vi "Draw parallelity.vi"(0 "Image in":T2, 1 "Arc width":u32=1, 3 "Overlay type":string, 5 "Bounding rectangle array":cluster{"X":dbl, "Y":dbl}[](array[cluster]), 7 "Fixed overlay in":T1, 9 "Size factor":dbl, 11 "error in (no error)":errorcluster, 12 "Overlay color":u32(colorbox)=16711680, 14 "Measurment Name":string) -> (4 "Image Out":T2, 6 "Overlay coordinates":cluster{"X":dbl, "Y":dbl}[](array[cluster]), 15 "error out":errorcluster)   [LabVIEW 2019]
uses:
  <vilib>/vision/Image Controls.llb/IMAQ Image.ctl
  <vilib>/vision/NI_Vision_Development_Module.lvlib
panel:
  in  "Array of input":string[](array[string])
  out "Offset height":dbl
  out "Offset width":dbl
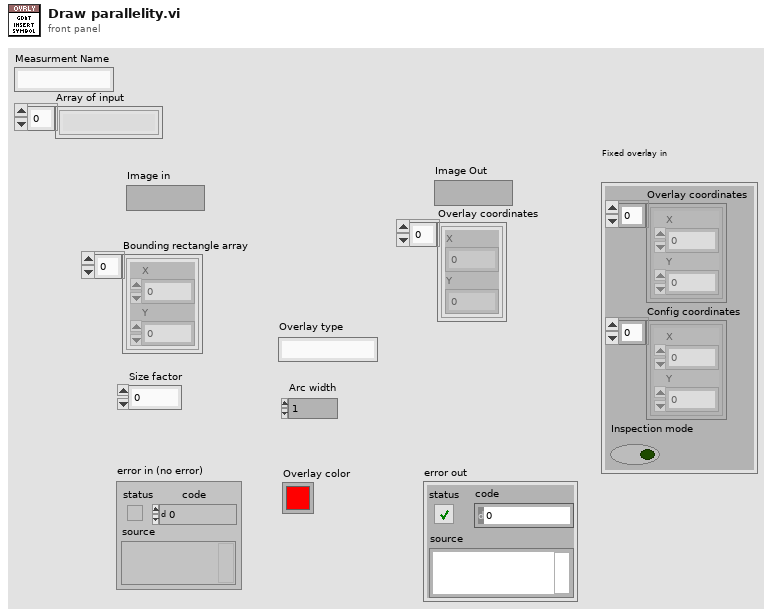
[diagram p1: front panel]
types:
  T1 = cluster{"Overlay coordinates":cluster{"X":dbl, "Y":dbl}[], "Config coordinates":cluster{"X":dbl, "Y":dbl}[], "Inspection mode":bool}
  T2 = typedef "IMAQ Image.ctl" = refnum<image>
  T3 = cluster{"Point 1":cluster{"X":sgl, "Y":sgl}, "Point 2":cluster{"X":sgl, "Y":sgl}}
  T4 = cluster{"Left":i32, "Top":i32, "Right":i32, "Bottom":i32}
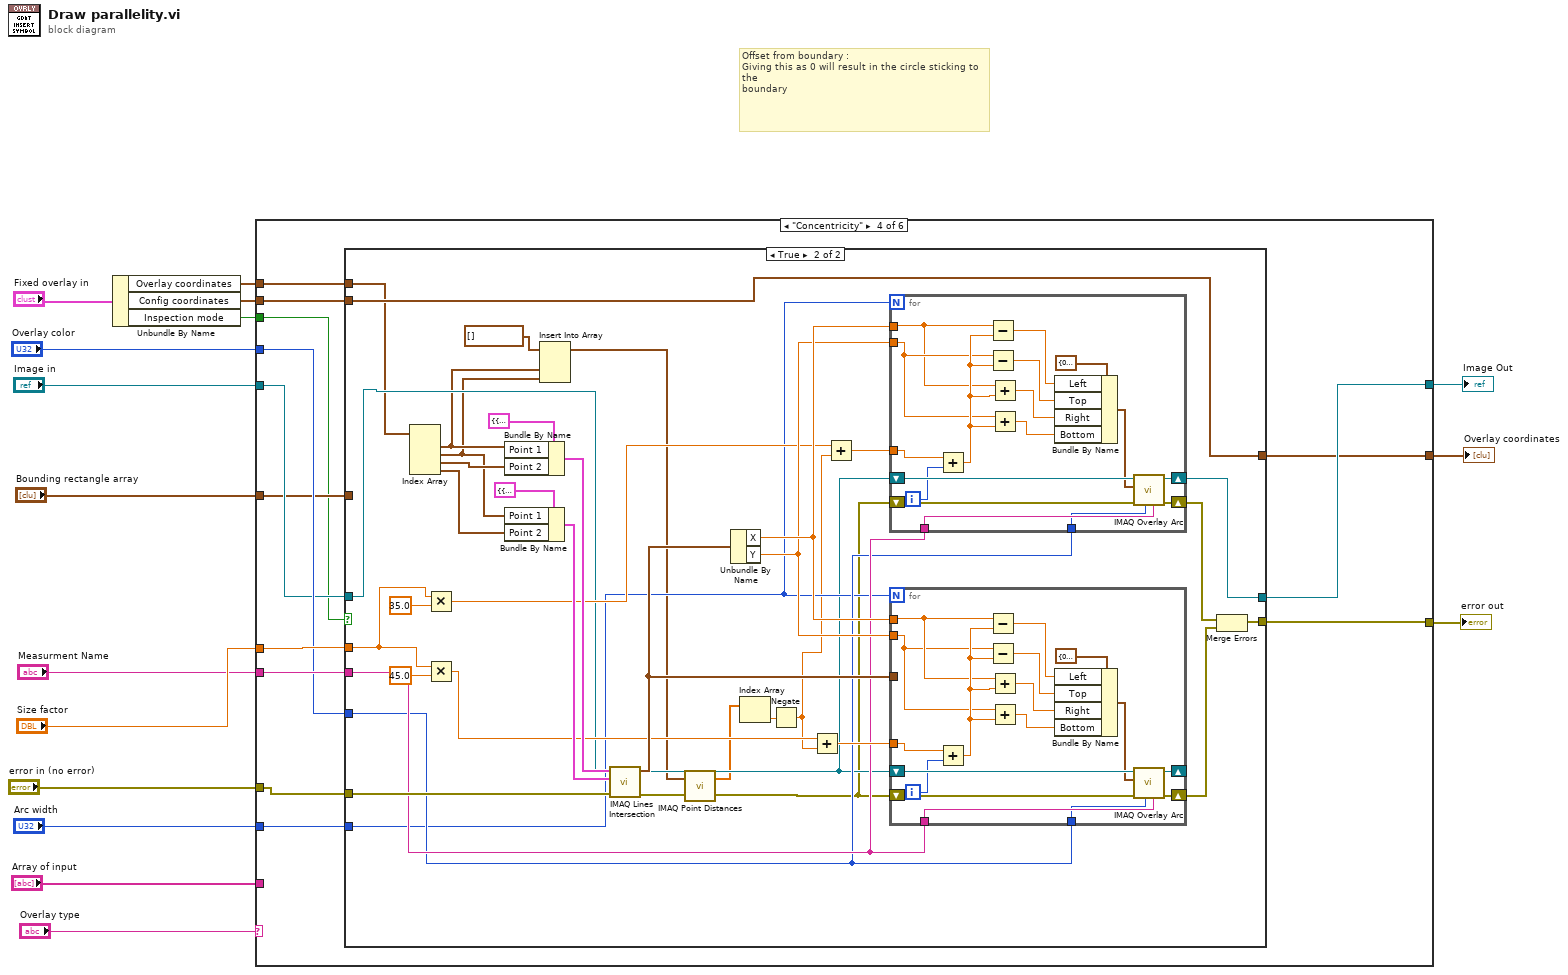
[diagram p0: block diagram]
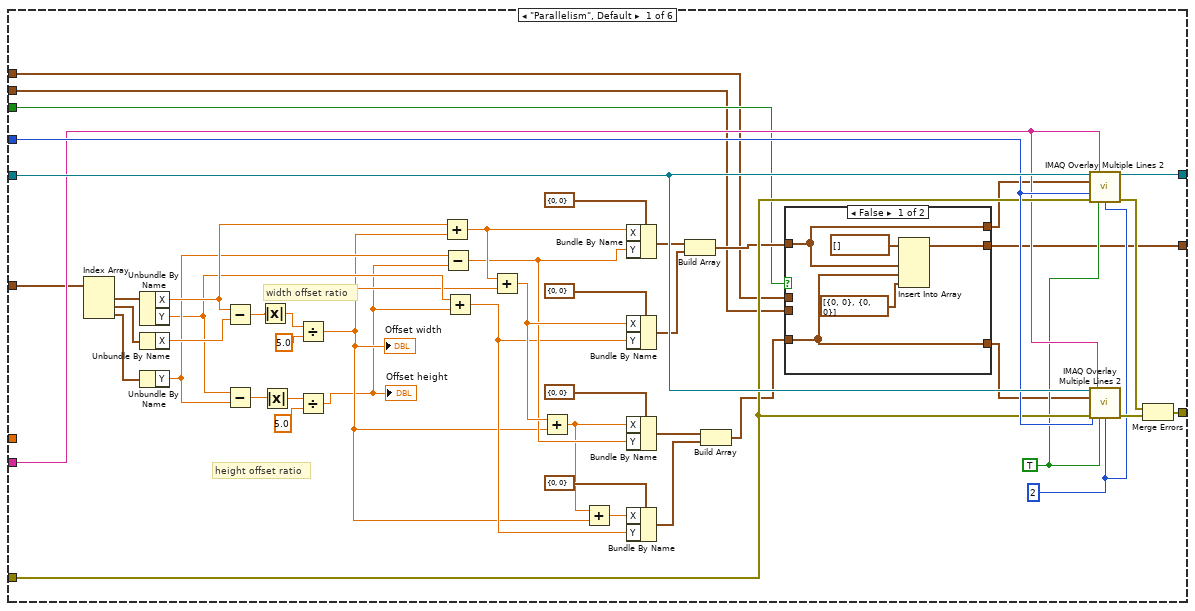
[diagram p2: hidden frame]
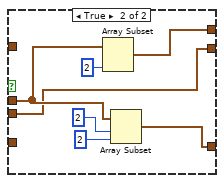
[diagram p3: hidden frame]
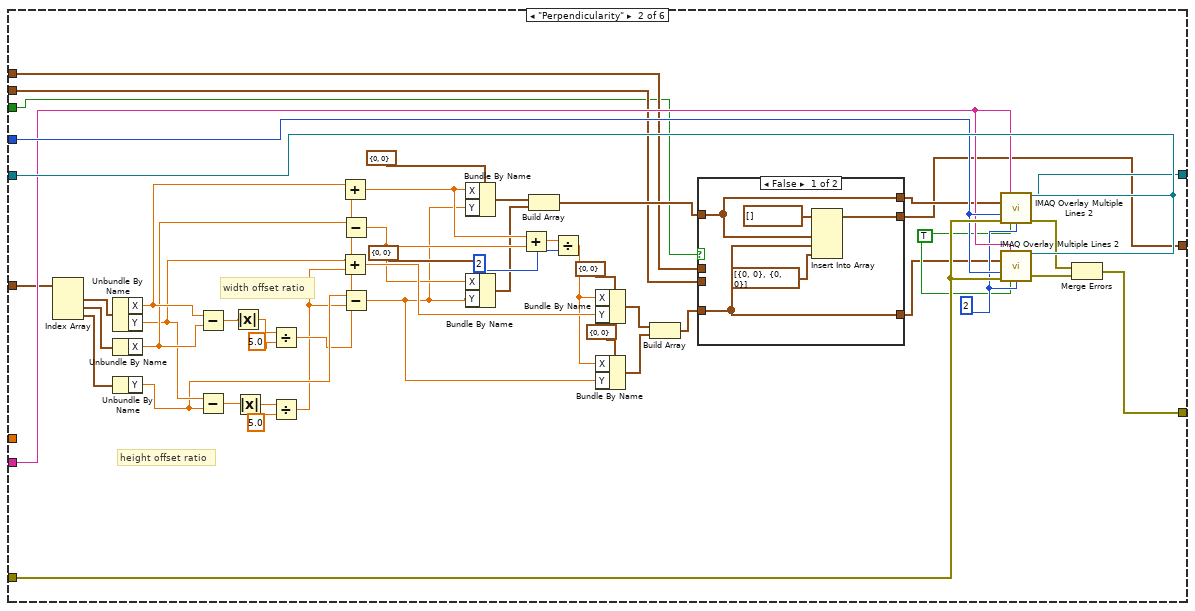
[diagram p4: hidden frame]
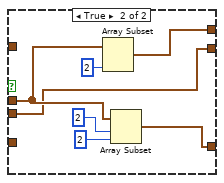
[diagram p5: hidden frame]
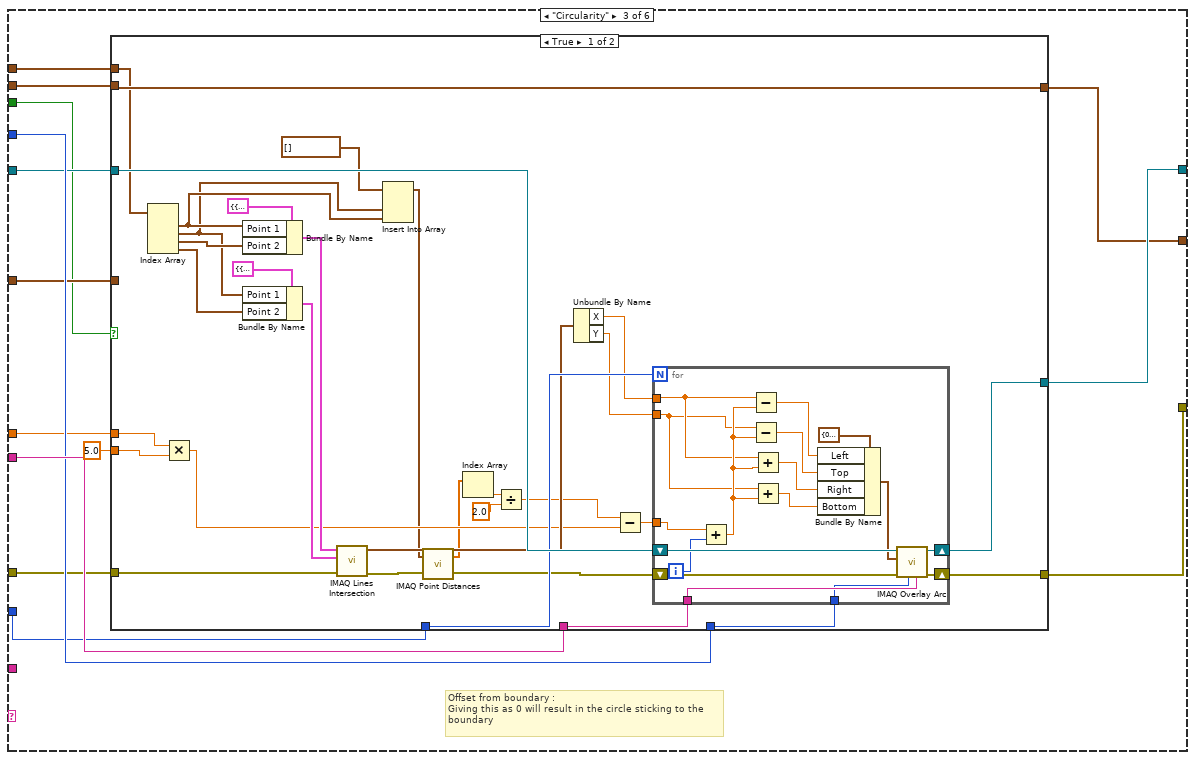
[diagram p6: hidden frame]
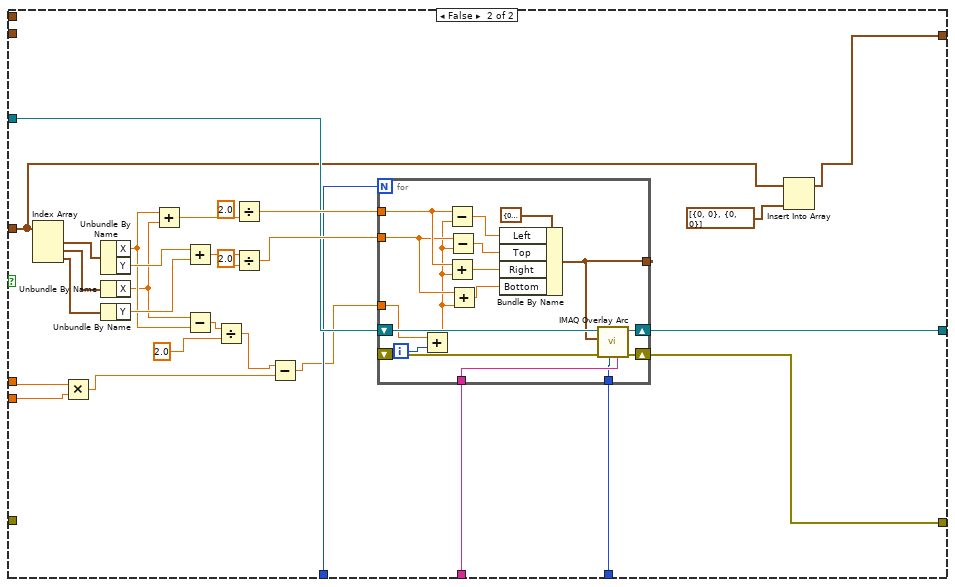
[diagram p7: hidden frame]
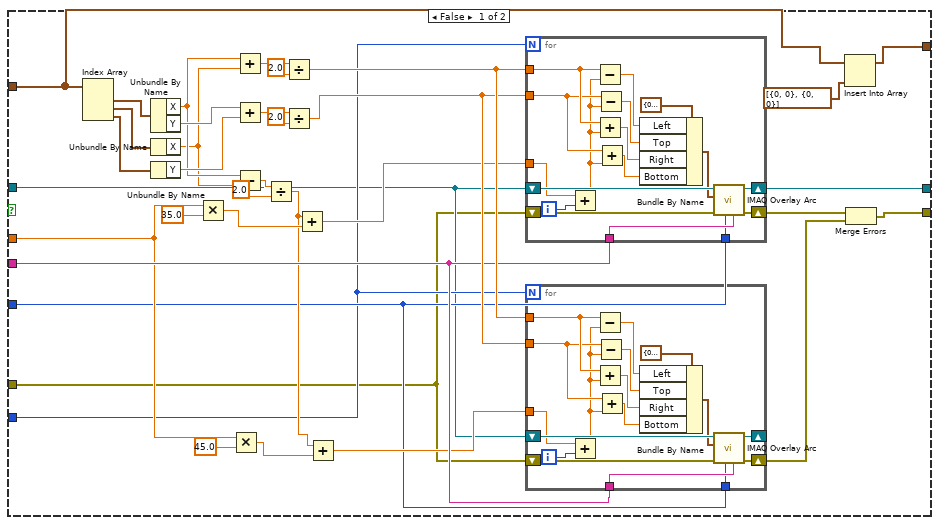
[diagram p8: hidden frame]
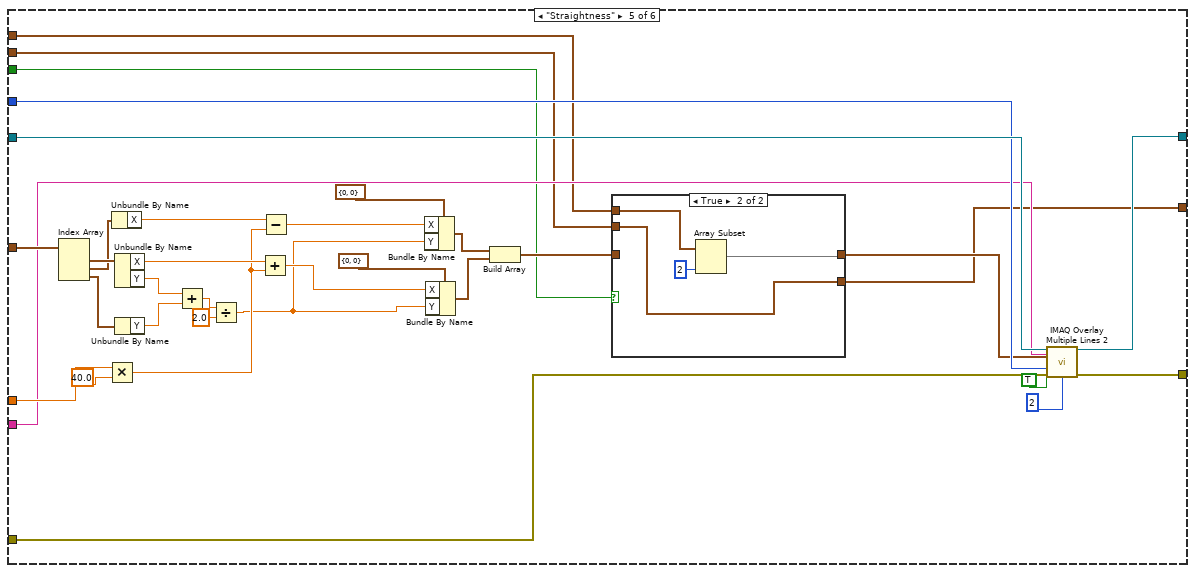
[diagram p9: hidden frame]
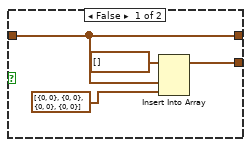
[diagram p10: hidden frame]
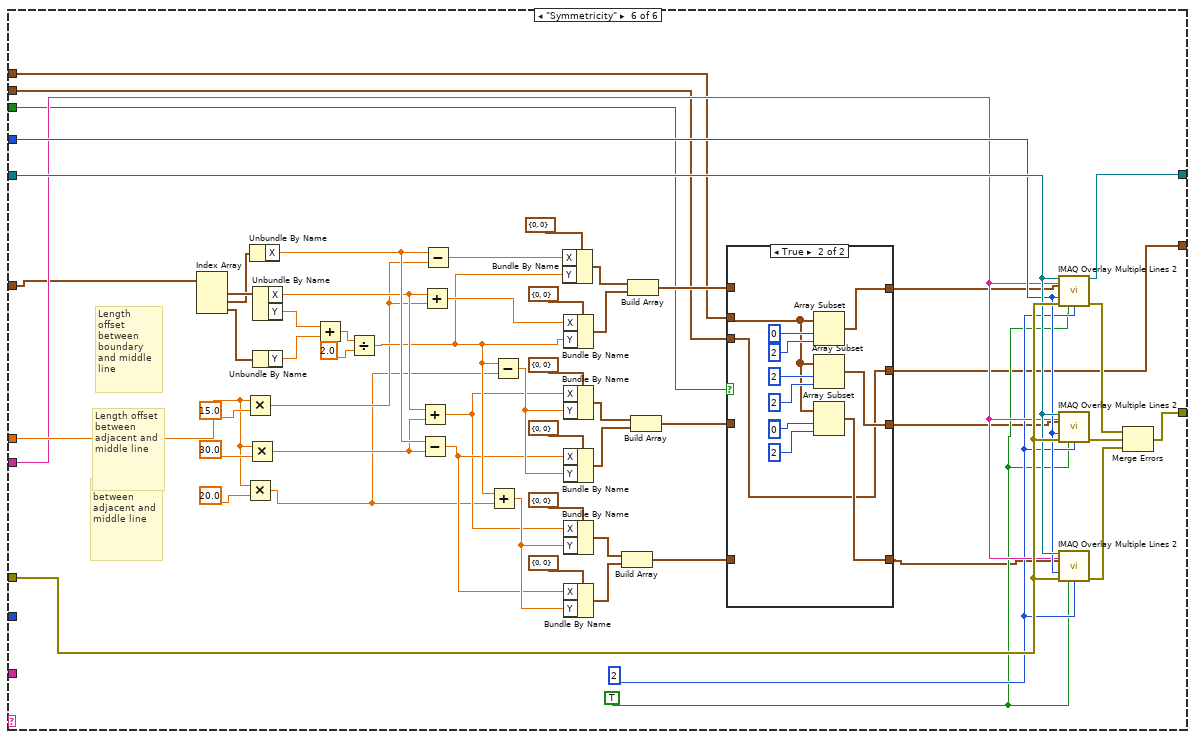
[diagram p11: hidden frame]
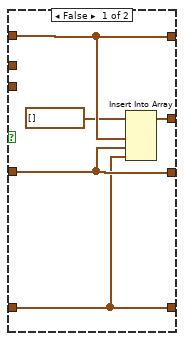
[diagram p12: hidden frame]
diagram:
  # "Offset from boundary :\nGiving this as 0 will result in the circle sticking to the\nboundary"
  n1 = Unbundle By Name("Fixed overlay in") -> ("Overlay coordinates"=w4:cluster{"X":dbl, "Y":dbl}[], "Config coordinates"=w3:cluster{"X":dbl, "Y":dbl}[], "Inspection mode"=w2:bool)
  n2 = case shown="\"Concentricity\"" "Overlay type" {
    tunnel: "Bounding rectangle array" -> [w25 w85 w144 w252 w429 w451]
    tunnel: "Size factor" -> [_ _ w146 w256 w424 w458]
    tunnel: "Image in" -> [w41 w98 w147 w253 w412 w463]
    tunnel: [w38 w94 w149 w259 w409 w455] -> w14
    tunnel: [w37 w93 w148 w258 w408 w483] -> w13
    tunnel: "Overlay color" -> [w36 w92 w150 w255 w411 w462]
    tunnel: "error in (no error)" -> [w31 w97 w140 w251 w410 w464]
    tunnel: "Arc width" -> [_ _ w145 w254 _ _]
    tunnel: "Measurment Name" -> [w28 w88 w151 w257 w407 w454]
    tunnel: "Array of input" -> [_ _ _ _ _ _]
    tunnel: w4 -> [w19 w79 w142 w248 w401 w443]
    tunnel: w3 -> [w18 w78 w143 w250 w400 w442]
    tunnel: w2 -> [w20 w77 w141 w247 w399 w444]
    tunnel: [w17 w80 w139 w249 w402 w441] -> w1
    frame "Parallelism", Default {
      w26 = u32 2 ("Width")
      w27 = TRUE ("Maintain Width?")
      # "height offset ratio"
      # "width offset ratio"
      n3 = Index Array(array=w25) -> (element #1=w64:cluster{"X":dbl, "Y":dbl}, element #2=w63:cluster{"X":dbl, "Y":dbl}, element #3=w58:cluster{"X":dbl, "Y":dbl})  [unwired: 3 in]
      n4 = Unbundle By Name(w64) -> ("X"=w53:dbl, "Y"=w49:dbl)
      n5 = Unbundle By Name(w63) -> ("X"=w62:dbl)
      n6 = Unbundle By Name(w58) -> ("Y"=w52:dbl)
      n7 = Subtract(x=w53, y=w62) -> (x-y=w60:dbl)
      n8 = Subtract(x=w49, y=w52) -> (x-y=w57:dbl)
      n9 = Absolute Value(x=w60) -> (abs(x)=w59:dbl)
      n10 = Absolute Value(x=w57) -> (abs(x)=w56:dbl)
      n11 = Divide(x=w59, y=5.0) -> (x/y=w30:dbl)
      "Offset width" <- w30
      n12 = Divide(x=w56, y=5.0) -> (x/y=w29:dbl)
      "Offset height" <- w29
      n13 = Add(x=w53, y=w30) -> (x+y=w50:dbl)
      n14 = Subtract(x=w52, y=w29) -> (x-y=w45:dbl)
      n15 = Add(x=w49, y=w29) -> (x+y=w42:dbl)
      n16 = Add(x=w50, y=w30) -> (x+y=w46:dbl)
      n17 = Add(x=w46, y=w30) -> (x+y=w43:dbl)
      n18 = Add(x=w43, y=w30) -> (x+y=w44:dbl)
      n19 = Bundle By Name(cluster=cluster{"X":i32, "Y":i32} {"X"=0, "Y"=0} ("Start Point"), "X"=w50, "Y"=w45) -> (w33:cluster{"X":i32, "Y":i32})
      n20 = Bundle By Name(cluster=cluster{"X":i32, "Y":i32} {"X"=0, "Y"=0} ("Start Point"), "X"=w46, "Y"=w42) -> (w32:cluster{"X":i32, "Y":i32})
      n21 = Bundle By Name(cluster=cluster{"X":i32, "Y":i32} {"X"=0, "Y"=0} ("Start Point"), "X"=w43, "Y"=w45) -> (w35:cluster{"X":i32, "Y":i32})
      n22 = Bundle By Name(cluster=cluster{"X":i32, "Y":i32} {"X"=0, "Y"=0} ("Start Point"), "X"=w44, "Y"=w42) -> (w34:cluster{"X":i32, "Y":i32})
      n23 = Build Array(w33, w32) -> (w24:cluster{"X":i32, "Y":i32}[])
      n24 = Build Array(w35, w34) -> (w22:cluster{"X":i32, "Y":i32}[])
      n25 = case shown="False" w20 {
        tunnel: w24 -> [w68 _]
        tunnel: w22 -> [w66 _]
        tunnel: [w68 w73] -> w23
        tunnel: [w67 w70] -> w17
        tunnel: [w66 w72] -> w21
        tunnel: w19 -> [_ w71]
        tunnel: w18 -> [_ w70]
        frame False {
          n26 = Insert Into Array(array=cluster{"X":i32, "Y":i32}[] [], new element #1=w68, new element #2=w66, new element #3=cluster{"X":i32, "Y":i32}[] [{"X"=0, "Y"=0}, {"X"=0, "Y"=0}]) -> (w67:cluster{"X":i32, "Y":i32}[])  [unwired: 1 in]
        }
        frame True {
          n27 = Array Subset(array=w71, length=2) -> (w73:cluster{"X":dbl, "Y":dbl}[])  [unwired: 1 in]
          n28 = Array Subset(array=w71, index=2 ("length"), length=2) -> (w72:cluster{"X":dbl, "Y":dbl}[])
        }
      }
      n29 = call "IMAQ Overlay Multiple Lines 2"("Image"=w41, "Group"=w28, "Line End Points"=w23, "Color"=w36, "error in (no error)"=w31, "Maintain Width?"=w27, "Width"=w26) -> ("Image Out"=w37:T2, "error out"=w40:errorcluster)  [unwired: 7 in]
      n30 = call "IMAQ Overlay Multiple Lines 2"("Image"=w41, "Group"=w28, "Line End Points"=w21, "Color"=w36, "error in (no error)"=w31, "Maintain Width?"=w27, "Width"=w26) -> ("error out"=w39:errorcluster)  [unwired: 7 in, 1 out]
      n31 = Merge Errors(w40, w39) -> (w38:errorcluster)
    }
    frame "Perpendicularity" {
      w87 = u32 2 ("Width")
      w86 = TRUE ("Maintain Width?")
      # "height offset ratio"
      # "width offset ratio"
      n32 = Index Array(array=w85) -> (element #1=w119:cluster{"X":dbl, "Y":dbl}, element #2=w118:cluster{"X":dbl, "Y":dbl}, element #3=w117:cluster{"X":dbl, "Y":dbl})  [unwired: 3 in]
      n33 = Unbundle By Name(w119) -> ("X"=w116:dbl, "Y"=w114:dbl)
      n34 = Unbundle By Name(w118) -> ("X"=w115:dbl)
      n35 = Unbundle By Name(w117) -> ("Y"=w91:dbl)
      n36 = Subtract(x=w116, y=w115) -> (x-y=w124:dbl)
      n37 = Subtract(x=w114, y=w91) -> (x-y=w122:dbl)
      n38 = Absolute Value(x=w124) -> (abs(x)=w123:dbl)
      n39 = Absolute Value(x=w122) -> (abs(x)=w121:dbl)
      n40 = Divide(x=w123, y=5.0) -> (x/y=w90:dbl)
      n41 = Divide(x=w121, y=5.0) -> (x/y=w89:dbl)
      n42 = Add(x=w116, y=w90) -> (x+y=w107:dbl)
      n43 = Add(x=w114, y=w89) -> (x+y=w110:dbl)
      n44 = Subtract(x=w115, y=w90) -> (x-y=w106:dbl)
      n45 = Subtract(x=w91, y=w89) -> (x-y=w103:dbl)
      n46 = Bundle By Name(cluster=cluster{"X":i32, "Y":i32} {"X"=0, "Y"=0} ("Start Point"), "X"=w107, "Y"=w103) -> (w102:cluster{"X":i32, "Y":i32})
      n47 = Bundle By Name(cluster=cluster{"X":i32, "Y":i32} {"X"=0, "Y"=0} ("Start Point"), "X"=w106, "Y"=w103) -> (w101:cluster{"X":i32, "Y":i32})
      n48 = Add(x=w107, y=w106) -> (x+y=w109:dbl)
      n49 = Build Array(w102, w101) -> (w82:cluster{"X":i32, "Y":i32}[])
      n50 = Divide(x=w109, y=2) -> (x/y=w104:dbl)
      n51 = Bundle By Name(cluster=cluster{"X":i32, "Y":i32} {"X"=0, "Y"=0} ("Start Point"), "X"=w104, "Y"=w110) -> (w100:cluster{"X":i32, "Y":i32})
      n52 = Bundle By Name(cluster=cluster{"X":i32, "Y":i32} {"X"=0, "Y"=0} ("Start Point"), "X"=w104, "Y"=w103) -> (w99:cluster{"X":i32, "Y":i32})
      n53 = Build Array(w100, w99) -> (w84:cluster{"X":i32, "Y":i32}[])
      n54 = case shown="False" w77 {
        tunnel: w82 -> [w129 _]
        tunnel: w84 -> [w127 _]
        tunnel: [w129 w134] -> w81
        tunnel: [w128 w131] -> w80
        tunnel: [w127 w133] -> w83
        tunnel: w79 -> [_ w132]
        tunnel: w78 -> [_ w131]
        frame False {
          n55 = Insert Into Array(array=cluster{"X":i32, "Y":i32}[] [], new element #1=w129, new element #2=w127, new element #3=cluster{"X":i32, "Y":i32}[] [{"X"=0, "Y"=0}, {"X"=0, "Y"=0}]) -> (w128:cluster{"X":i32, "Y":i32}[])  [unwired: 1 in]
        }
        frame True {
          n56 = Array Subset(array=w132, length=2) -> (w134:cluster{"X":dbl, "Y":dbl}[])  [unwired: 1 in]
          n57 = Array Subset(array=w132, index=2 ("length"), length=2) -> (w133:cluster{"X":dbl, "Y":dbl}[])
        }
      }
      n58 = call "IMAQ Overlay Multiple Lines 2"("Image"=w98, "Group"=w88, "Line End Points"=w81, "Color"=w92, "error in (no error)"=w97, "Maintain Width?"=w86, "Width"=w87) -> ("Image Out"=w93:T2, "error out"=w95:errorcluster)  [unwired: 7 in]
      n59 = call "IMAQ Overlay Multiple Lines 2"("Image"=w98, "Group"=w88, "Line End Points"=w83, "Color"=w92, "error in (no error)"=w97, "Maintain Width?"=w86, "Width"=w87) -> ("error out"=w96:errorcluster)  [unwired: 7 in, 1 out]
      n60 = Merge Errors(w95, w96) -> (w94:errorcluster)
    }
    frame "Circularity" {
      # "Offset from boundary :\nGiving this as 0 will result in the circle sticking to the\nboundary"
      n61 = case shown="True" w141 {
        tunnel: w151 -> [w183 w215]
        tunnel: w150 -> [w182 w214]
        tunnel: [w181 w213] -> w149
        tunnel: [w180 w212] -> w148
        tunnel: w147 -> [w179 w211]
        tunnel: w146 -> [w165 w205]
        tunnel: w145 -> [w178 w209]
        tunnel: w144 -> [_ w207]
        tunnel: [w177 w206] -> w139
        tunnel: w143 -> [w177 _]
        tunnel: w142 -> [w176 _]
        tunnel: w140 -> [w171 _]
        tunnel: 5.0 ("y") -> [w162 w201]
        frame True {
          n62 = Index Array(array=w176) -> (element #1=w160:cluster{"X":dbl, "Y":dbl}, element #2=w159:cluster{"X":dbl, "Y":dbl}, element #3=w173:cluster{"X":dbl, "Y":dbl}, element #4=w172:cluster{"X":dbl, "Y":dbl})  [unwired: 4 in]
          n63 = Multiply(x=w165, y=w162) -> (x*y=w164:dbl)
          n64 = Bundle By Name(cluster=T3 {"Point 1"={"X"=0.0, "Y"=0.0}, "Point 2"={"X"=0.0, "Y"=0.0}} ("Line 1"), "Point 1"=w160, "Point 2"=w173) -> (w170:T3)
          n65 = Bundle By Name(cluster=T3 {"Point 1"={"X"=0.0, "Y"=0.0}, "Point 2"={"X"=0.0, "Y"=0.0}} ("Line 1"), "Point 1"=w159, "Point 2"=w172) -> (w169:T3)
          n66 = call "IMAQ Lines Intersection"("error in (no error)"=w171, "Line 2"=w169, "Line 1"=w170) -> ("error out"=w161:errorcluster, "Intersection Point"=w166:cluster{"X":sgl, "Y":sgl})  [unwired: 6 in, 1 out]
          n67 = Insert Into Array(array=cluster{"X":dbl, "Y":dbl}[] [], new element #1=w159, new element #2=w160) -> (w157:cluster{"X":dbl, "Y":dbl}[])  [unwired: 1 in]
          n68 = call "IMAQ Point Distances"("Points"=w157, "error in (no error)"=w161) -> ("Distances"=w156:sgl[], "error out"=w152:errorcluster)  [unwired: 3 in]
          n69 = Index Array(array=w156) -> (element=w155:sgl)  [unwired: 1 in]
          n70 = Divide(x=w155, y=sgl 2.0) -> (x/y=w153:sgl)
          n71 = Unbundle By Name(w166) -> ("X"=w168:sgl, "Y"=w167:sgl)
          n72 = Subtract(x=w153, y=w164) -> (x-y=w163:dbl)
          n73 = for {
            N: w178 -> [_]
            shift-right: [w199] -> w181
            shift-left: w152 -> [w200]
            shift-right: [w197] -> w180
            shift-left: w179 -> [w198]
            tunnel: w183 -> [w195]
            tunnel: w182 -> [w194]
            tunnel: w168 -> [w185]
            tunnel: w167 -> [w184]
            tunnel: w163 -> [w188]
            i -> [w187]
            n74 = Add(x=w188, y=w187) -> (x+y=w186:dbl)
            n75 = Subtract(x=w185, y=w186) -> (x-y=w192:dbl)
            n76 = Subtract(x=w184, y=w186) -> (x-y=w191:dbl)
            n77 = Add(x=w185, y=w186) -> (x+y=w190:dbl)
            n78 = Add(x=w184, y=w186) -> (x+y=w189:dbl)
            n79 = Bundle By Name(cluster=T4 {"Left"=0, "Top"=0, "Right"=0, "Bottom"=0} ("Bounding Rectangle"), "Left"=w192, "Top"=w191, "Right"=w190, "Bottom"=w189) -> (w193:T4)
            n80 = call "IMAQ Overlay Arc"("Group"=w195, "Color"=w194, "error in (no error)"=w200, "Bounding Rectangle"=w193, "Image"=w198) -> ("error out"=w199:errorcluster, "Image Out"=w197:T2)  [unwired: 5 in]
          }
        }
        frame False {
          n81 = Index Array(array=w207) -> (element #1=w229:cluster{"X":dbl, "Y":dbl}, element #2=w228:cluster{"X":dbl, "Y":dbl}, element #3=w227:cluster{"X":dbl, "Y":dbl})  [unwired: 3 in]
          n82 = Multiply(x=w205, y=w201) -> (x*y=w203:dbl)
          n83 = Unbundle By Name(w229) -> ("X"=w218:dbl, "Y"=w222:dbl)
          n84 = Unbundle By Name(w228) -> ("X"=w217:dbl)
          n85 = Unbundle By Name(w227) -> ("Y"=w221:dbl)
          n86 = Add(x=w218, y=w217) -> (x+y=w226:dbl)
          n87 = Add(x=w222, y=w221) -> (x+y=w223:dbl)
          n88 = Subtract(x=w217, y=w218) -> (x-y=w216:dbl)
          n89 = Divide(x=w216, y=2.0) -> (x/y=w204:dbl)
          n90 = Divide(x=w226, y=2.0) -> (x/y=w220:dbl)
          n91 = Divide(x=w223, y=2.0) -> (x/y=w219:dbl)
          n92 = Subtract(x=w204, y=w203) -> (x-y=w202:dbl)
          n93 = for {
            N: w209 -> [_]
            tunnel: w220 -> [w239]
            tunnel: w219 -> [w237]
            tunnel: w202 -> [w234]
            shift-right: [w245] -> w213
            shift-left: _ -> [w246]
            shift-right: [w243] -> w212
            shift-left: w211 -> [w244]
            tunnel: w215 -> [w232]
            tunnel: w214 -> [w231]
            tunnel: [w230] -> _
            i -> [w235]
            n94 = Add(x=w234, y=w235) -> (x+y=w233:dbl)
            n95 = Subtract(x=w239, y=w233) -> (x-y=w241:dbl)
            n96 = Add(x=w239, y=w233) -> (x+y=w238:dbl)
            n97 = Subtract(x=w237, y=w233) -> (x-y=w240:dbl)
            n98 = Add(x=w237, y=w233) -> (x+y=w236:dbl)
            n99 = Bundle By Name(cluster=T4 {"Left"=0, "Top"=0, "Right"=0, "Bottom"=0} ("Bounding Rectangle"), "Left"=w241, "Top"=w240, "Right"=w238, "Bottom"=w236) -> (w230:T4)
            n100 = call "IMAQ Overlay Arc"("Group"=w232, "Color"=w231, "error in (no error)"=w246, "Bounding Rectangle"=w230, "Image"=w244) -> ("error out"=w245:errorcluster, "Image Out"=w243:T2)  [unwired: 5 in]
          }
          n101 = Insert Into Array(array=w207, new element=cluster{"X":i32, "Y":i32}[] [{"X"=0, "Y"=0}, {"X"=0, "Y"=0}]) -> (w206:cluster{"X":dbl, "Y":dbl}[])  [unwired: 1 in]
        }
      }
    }
    frame "Concentricity" {
      n102 = case shown="True" w247 {
        tunnel: [w264 w354] -> w259
        tunnel: [w282 w341] -> w258
        tunnel: w257 -> [w275 w344]
        tunnel: w256 -> [w272 w347]
        tunnel: w255 -> [w269 w343]
        tunnel: w254 -> [w268 w342]
        tunnel: w253 -> [w267 w340]
        tunnel: w252 -> [w261 _]
        tunnel: w251 -> [w263 w355]
        tunnel: w250 -> [_ w339]
        tunnel: [w260 w339] -> w249
        tunnel: w248 -> [_ w338]
        frame False {
          n103 = Index Array(array=w261) -> (element #1=w294:cluster{"X":dbl, "Y":dbl}, element #2=w293:cluster{"X":dbl, "Y":dbl}, element #3=w292:cluster{"X":dbl, "Y":dbl})  [unwired: 3 in]
          n104 = Unbundle By Name(w294) -> ("X"=w285:dbl, "Y"=w287:dbl)
          n105 = Unbundle By Name(w293) -> ("X"=w284:dbl)
          n106 = Unbundle By Name(w292) -> ("Y"=w286:dbl)
          n107 = Multiply(x=w272, y=35.0) -> (x*y=w279:dbl)
          n108 = Multiply(x=w272, y=45.0) -> (x*y=w271:dbl)
          n109 = Add(x=w285, y=w284) -> (x+y=w291:dbl)
          n110 = Add(x=w287, y=w286) -> (x+y=w288:dbl)
          n111 = Subtract(x=w285, y=w284) -> (x-y=w283:dbl)
          n112 = Divide(x=w283, y=2.0) -> (x/y=w274:dbl)
          n113 = Divide(x=w291, y=2.0) -> (x/y=w278:dbl)
          n114 = Divide(x=w288, y=2.0) -> (x/y=w277:dbl)
          n115 = Add(x=w274, y=w279) -> (x+y=w276:dbl)
          n116 = Add(x=w274, y=w271) -> (x+y=w270:dbl)
          n117 = for {
            N: w268 -> [_]
            tunnel: w278 -> [w320]
            tunnel: w277 -> [w318]
            tunnel: w276 -> [w315]
            shift-right: [w327] -> w266
            shift-left: w263 -> [w328]
            shift-right: [w325] -> w282
            shift-left: w267 -> [w326]
            tunnel: w275 -> [w313]
            tunnel: w269 -> [w312]
            i -> [w316]
            n118 = Add(x=w315, y=w316) -> (x+y=w314:dbl)
            n119 = Subtract(x=w320, y=w314) -> (x-y=w322:dbl)
            n120 = Add(x=w320, y=w314) -> (x+y=w319:dbl)
            n121 = Subtract(x=w318, y=w314) -> (x-y=w321:dbl)
            n122 = Add(x=w318, y=w314) -> (x+y=w317:dbl)
            n123 = Bundle By Name(cluster=T4 {"Left"=0, "Top"=0, "Right"=0, "Bottom"=0} ("Bounding Rectangle"), "Left"=w322, "Top"=w321, "Right"=w319, "Bottom"=w317) -> (w323:T4)
            n124 = call "IMAQ Overlay Arc"("Group"=w313, "Color"=w312, "error in (no error)"=w328, "Bounding Rectangle"=w323, "Image"=w326) -> ("error out"=w327:errorcluster, "Image Out"=w325:T2)  [unwired: 5 in]
          }
          n125 = for {
            N: w268 -> [_]
            tunnel: w278 -> [w303]
            tunnel: w277 -> [w301]
            tunnel: w270 -> [w298]
            shift-right: [w310] -> w265
            shift-left: w263 -> [w311]
            shift-right: [w308] -> _
            shift-left: w267 -> [w309]
            tunnel: w275 -> [w296]
            tunnel: w269 -> [w295]
            i -> [w299]
            n126 = Add(x=w298, y=w299) -> (x+y=w297:dbl)
            n127 = Subtract(x=w303, y=w297) -> (x-y=w305:dbl)
            n128 = Add(x=w303, y=w297) -> (x+y=w302:dbl)
            n129 = Subtract(x=w301, y=w297) -> (x-y=w304:dbl)
            n130 = Add(x=w301, y=w297) -> (x+y=w300:dbl)
            n131 = Bundle By Name(cluster=T4 {"Left"=0, "Top"=0, "Right"=0, "Bottom"=0} ("Bounding Rectangle"), "Left"=w305, "Top"=w304, "Right"=w302, "Bottom"=w300) -> (w306:T4)
            n132 = call "IMAQ Overlay Arc"("Group"=w296, "Color"=w295, "error in (no error)"=w311, "Bounding Rectangle"=w306, "Image"=w309) -> ("error out"=w310:errorcluster, "Image Out"=w308:T2)  [unwired: 5 in]
          }
          n133 = Insert Into Array(array=w261, new element=cluster{"X":i32, "Y":i32}[] [{"X"=0, "Y"=0}, {"X"=0, "Y"=0}]) -> (w260:cluster{"X":dbl, "Y":dbl}[])  [unwired: 1 in]
          n134 = Merge Errors(w266, w265) -> (w264:errorcluster)
        }
        frame True {
          n135 = Index Array(array=w338) -> (element #1=w335:cluster{"X":dbl, "Y":dbl}, element #2=w334:cluster{"X":dbl, "Y":dbl}, element #3=w362:cluster{"X":dbl, "Y":dbl}, element #4=w361:cluster{"X":dbl, "Y":dbl})  [unwired: 4 in]
          n136 = Multiply(x=w347, y=35.0) -> (x*y=w346:dbl)
          n137 = Multiply(x=w347, y=45.0) -> (x*y=w356:dbl)
          n138 = Bundle By Name(cluster=T3 {"Point 1"={"X"=0.0, "Y"=0.0}, "Point 2"={"X"=0.0, "Y"=0.0}} ("Line 1"), "Point 1"=w335, "Point 2"=w362) -> (w360:T3)
          n139 = Bundle By Name(cluster=T3 {"Point 1"={"X"=0.0, "Y"=0.0}, "Point 2"={"X"=0.0, "Y"=0.0}} ("Line 1"), "Point 1"=w334, "Point 2"=w361) -> (w359:T3)
          n140 = Insert Into Array(array=cluster{"X":dbl, "Y":dbl}[] [], new element #1=w335, new element #2=w334) -> (w332:cluster{"X":dbl, "Y":dbl}[])  [unwired: 1 in]
          n141 = call "IMAQ Lines Intersection"("error in (no error)"=w355, "Line 2"=w359, "Line 1"=w360) -> ("error out"=w337:errorcluster, "Intersection Point"=w358:cluster{"X":sgl, "Y":sgl})  [unwired: 6 in, 1 out]
          n142 = call "IMAQ Point Distances"("Points"=w332, "error in (no error)"=w337) -> ("Distances"=w331:sgl[], "error out"=w336:errorcluster)  [unwired: 3 in]
          n143 = Unbundle By Name(w358) -> ("X"=w351:sgl, "Y"=w350:sgl)
          n144 = Index Array(array=w331) -> (element=w330:sgl)  [unwired: 1 in]
          n145 = Negate(x=w330) -> (-x=w329:sgl)
          n146 = Add(x=w356, y=w329) -> (x+y=w349:dbl)
          n147 = Add(x=w346, y=w329) -> (x+y=w345:dbl)
          n148 = for {
            N: w342 -> [_]
            shift-right: [w380] -> w352
            shift-left: w336 -> [w381]
            shift-right: [w378] -> w341
            shift-left: w340 -> [w379]
            tunnel: w344 -> [w376]
            tunnel: w343 -> [w375]
            tunnel: w351 -> [w365]
            tunnel: w350 -> [w366]
            tunnel: w345 -> [w369]
            i -> [w368]
            n149 = Add(x=w369, y=w368) -> (x+y=w367:dbl)
            n150 = Subtract(x=w365, y=w367) -> (x-y=w373:dbl)
            n151 = Subtract(x=w366, y=w367) -> (x-y=w372:dbl)
            n152 = Add(x=w365, y=w367) -> (x+y=w371:dbl)
            n153 = Add(x=w366, y=w367) -> (x+y=w370:dbl)
            n154 = Bundle By Name(cluster=T4 {"Left"=0, "Top"=0, "Right"=0, "Bottom"=0} ("Bounding Rectangle"), "Left"=w373, "Top"=w372, "Right"=w371, "Bottom"=w370) -> (w374:T4)
            n155 = call "IMAQ Overlay Arc"("Group"=w376, "Color"=w375, "error in (no error)"=w381, "Bounding Rectangle"=w374, "Image"=w379) -> ("error out"=w380:errorcluster, "Image Out"=w378:T2)  [unwired: 5 in]
          }
          n156 = for {
            N: w342 -> [_]
            shift-right: [w397] -> w353
            shift-left: w336 -> [w398]
            shift-right: [w395] -> _
            shift-left: w340 -> [w396]
            tunnel: w344 -> [w393]
            tunnel: w343 -> [w392]
            tunnel: w358 -> [_]
            tunnel: w351 -> [w383]
            tunnel: w350 -> [w382]
            tunnel: w349 -> [w386]
            i -> [w385]
            n157 = Add(x=w386, y=w385) -> (x+y=w384:dbl)
            n158 = Subtract(x=w383, y=w384) -> (x-y=w390:dbl)
            n159 = Subtract(x=w382, y=w384) -> (x-y=w389:dbl)
            n160 = Add(x=w383, y=w384) -> (x+y=w388:dbl)
            n161 = Add(x=w382, y=w384) -> (x+y=w387:dbl)
            n162 = Bundle By Name(cluster=T4 {"Left"=0, "Top"=0, "Right"=0, "Bottom"=0} ("Bounding Rectangle"), "Left"=w390, "Top"=w389, "Right"=w388, "Bottom"=w387) -> (w391:T4)
            n163 = call "IMAQ Overlay Arc"("Group"=w393, "Color"=w392, "error in (no error)"=w398, "Bounding Rectangle"=w391, "Image"=w396) -> ("error out"=w397:errorcluster, "Image Out"=w395:T2)  [unwired: 5 in]
          }
          n164 = Merge Errors(w352, w353) -> (w354:errorcluster)
        }
      }
    }
    frame "Straightness" {
      n165 = Index Array(array=w429) -> (element #1=w432:cluster{"X":dbl, "Y":dbl}, element #2=w431:cluster{"X":dbl, "Y":dbl}, element #3=w430:cluster{"X":dbl, "Y":dbl})  [unwired: 3 in]
      n166 = Multiply(x=w424, y=40.0) -> (x*y=w420:dbl)
      n167 = Unbundle By Name(w431) -> ("X"=w422:dbl)
      n168 = Unbundle By Name(w432) -> ("X"=w421:dbl, "Y"=w428:dbl)
      n169 = Unbundle By Name(w430) -> ("Y"=w427:dbl)
      n170 = Add(x=w428, y=w427) -> (x+y=w426:dbl)
      n171 = Divide(x=w426, y=2.0) -> (x/y=w415:dbl)
      n172 = Add(x=w421, y=w420) -> (x+y=w416:dbl)
      n173 = Subtract(x=w422, y=w420) -> (x-y=w417:dbl)
      n174 = Bundle By Name(cluster=cluster{"X":i32, "Y":i32} {"X"=0, "Y"=0} ("Start Point"), "X"=w417, "Y"=w415) -> (w414:cluster{"X":i32, "Y":i32})
      n175 = Bundle By Name(cluster=cluster{"X":i32, "Y":i32} {"X"=0, "Y"=0} ("Start Point"), "X"=w416, "Y"=w415) -> (w413:cluster{"X":i32, "Y":i32})
      n176 = Build Array(w414, w413) -> (w404:cluster{"X":i32, "Y":i32}[])
      n177 = case shown="True" w399 {
        tunnel: w404 -> [w436 _]
        tunnel: [w436 w438] -> w403
        tunnel: [w434 w437] -> w402
        tunnel: w401 -> [_ w440]
        tunnel: w400 -> [_ w437]
        frame False {
          n178 = Insert Into Array(array=cluster{"X":i32, "Y":i32}[] [], new element #1=w436, new element #2=cluster{"X":i32, "Y":i32}[] [{"X"=0, "Y"=0}, {"X"=0, "Y"=0}, {"X"=0, "Y"=0}, {"X"=0, "Y"=0}]) -> (w434:cluster{"X":i32, "Y":i32}[])  [unwired: 1 in]
        }
        frame True {
          n179 = Array Subset(array=w440, length=2) -> (w438:cluster{"X":dbl, "Y":dbl}[])  [unwired: 1 in]
        }
      }
      n180 = call "IMAQ Overlay Multiple Lines 2"("Image"=w412, "Group"=w407, "Line End Points"=w403, "Color"=w411, "error in (no error)"=w410, "Maintain Width?"=TRUE, "Width"=u32 2) -> ("Image Out"=w408:T2, "error out"=w409:errorcluster)  [unwired: 7 in]
    }
    frame "Symmetricity" {
      w453 = u32 2 ("Width")
      w452 = TRUE ("Maintain Width?")
      # "Height offset between adjacent and middle line"
      # "Length offset between adjacent and middle line"
      # "Length offset between boundary and middle line"
      n181 = Index Array(array=w451) -> (element #1=w497:cluster{"X":dbl, "Y":dbl}, element #2=w496:cluster{"X":dbl, "Y":dbl}, element #3=w495:cluster{"X":dbl, "Y":dbl})  [unwired: 3 in]
      n182 = Multiply(x=w458, y=15.0) -> (x*y=w474:dbl)
      n183 = Multiply(x=w458, y=20.0) -> (x*y=w456:dbl)
      n184 = Multiply(x=w458, y=30.0) -> (x*y=w479:dbl)
      n185 = Unbundle By Name(w496) -> ("X"=w481:dbl)
      n186 = Unbundle By Name(w497) -> ("X"=w480:dbl, "Y"=w494:dbl)
      n187 = Unbundle By Name(w495) -> ("Y"=w493:dbl)
      n188 = Add(x=w494, y=w493) -> (x+y=w492:dbl)
      n189 = Divide(x=w492, y=2.0) -> (x/y=w475:dbl)
      n190 = Add(x=w480, y=w479) -> (x+y=w469:dbl)
      n191 = Subtract(x=w481, y=w479) -> (x-y=w470:dbl)
      n192 = Add(x=w480, y=w474) -> (x+y=w486:dbl)
      n193 = Subtract(x=w481, y=w474) -> (x-y=w487:dbl)
      n194 = Add(x=w475, y=w456) -> (x+y=w471:dbl)
      n195 = Subtract(x=w475, y=w456) -> (x-y=w476:dbl)
      n196 = Bundle By Name(cluster=cluster{"X":i32, "Y":i32} {"X"=0, "Y"=0} ("Start Point"), "X"=w487, "Y"=w475) -> (w485:cluster{"X":i32, "Y":i32})
      n197 = Bundle By Name(cluster=cluster{"X":i32, "Y":i32} {"X"=0, "Y"=0} ("Start Point"), "X"=w486, "Y"=w475) -> (w484:cluster{"X":i32, "Y":i32})
      n198 = Bundle By Name(cluster=cluster{"X":i32, "Y":i32} {"X"=0, "Y"=0} ("Start Point"), "X"=w469, "Y"=w476) -> (w468:cluster{"X":i32, "Y":i32})
      n199 = Bundle By Name(cluster=cluster{"X":i32, "Y":i32} {"X"=0, "Y"=0} ("Start Point"), "X"=w470, "Y"=w476) -> (w467:cluster{"X":i32, "Y":i32})
      n200 = Bundle By Name(cluster=cluster{"X":i32, "Y":i32} {"X"=0, "Y"=0} ("Start Point"), "X"=w469, "Y"=w471) -> (w466:cluster{"X":i32, "Y":i32})
      n201 = Bundle By Name(cluster=cluster{"X":i32, "Y":i32} {"X"=0, "Y"=0} ("Start Point"), "X"=w470, "Y"=w471) -> (w465:cluster{"X":i32, "Y":i32})
      n202 = Build Array(w466, w465) -> (w446:cluster{"X":i32, "Y":i32}[])
      n203 = Build Array(w485, w484) -> (w449:cluster{"X":i32, "Y":i32}[])
      n204 = Build Array(w468, w467) -> (w447:cluster{"X":i32, "Y":i32}[])
      n205 = case shown="True" w444 {
        tunnel: [w502 w507] -> w450
        tunnel: w449 -> [w502 _]
        tunnel: [w501 w505] -> w448
        tunnel: w447 -> [w501 _]
        tunnel: w446 -> [w500 _]
        tunnel: [w500 w504] -> w445
        tunnel: w443 -> [_ w506]
        tunnel: w442 -> [_ w503]
        tunnel: [w498 w503] -> w441
        frame False {
          n206 = Insert Into Array(array=cluster{"X":i32, "Y":i32}[] [], new element #1=w502, new element #2=w501, new element #3=w500) -> (w498:cluster{"X":i32, "Y":i32}[])  [unwired: 1 in]
        }
        frame True {
          (unwired) 0 ("index")
          n207 = Array Subset(array=w506, index=0, length=2 ("index")) -> (w507:cluster{"X":dbl, "Y":dbl}[])
          n208 = Array Subset(array=w506, index=2, length=2 ("index")) -> (w505:cluster{"X":dbl, "Y":dbl}[])
          n209 = Array Subset(array=w506, index=4, length=2 ("index")) -> (w504:cluster{"X":dbl, "Y":dbl}[])
        }
      }
      n210 = call "IMAQ Overlay Multiple Lines 2"("Image"=w463, "Group"=w454, "Line End Points"=w450, "Color"=w462, "error in (no error)"=w464, "Maintain Width?"=w452, "Width"=w453) -> ("Image Out"=w483:T2, "error out"=w461:errorcluster)  [unwired: 7 in]
      n211 = call "IMAQ Overlay Multiple Lines 2"("Image"=w463, "Group"=w454, "Line End Points"=w448, "Color"=w462, "error in (no error)"=w464, "Maintain Width?"=w452, "Width"=w453) -> ("error out"=w460:errorcluster)  [unwired: 7 in, 1 out]
      n212 = call "IMAQ Overlay Multiple Lines 2"("Image"=w463, "Group"=w454, "Line End Points"=w445, "Color"=w462, "error in (no error)"=w464, "Maintain Width?"=w452, "Width"=w453) -> ("error out"=w459:errorcluster)  [unwired: 7 in, 1 out]
      n213 = Merge Errors(w461, w460, w459) -> (w455:errorcluster)
    }
  }
  "error out" <- w14
  "Image Out" <- w13
  "Overlay coordinates" <- w1
